vi "Get Functions Path.vi"(8 "error in (no error)":errorcluster) -> (0 "error out":errorcluster, 3 "Function List":path)   [LabVIEW 2016, in "scripts manager.lvclass"]
uses:
  scripts manager.lvclass
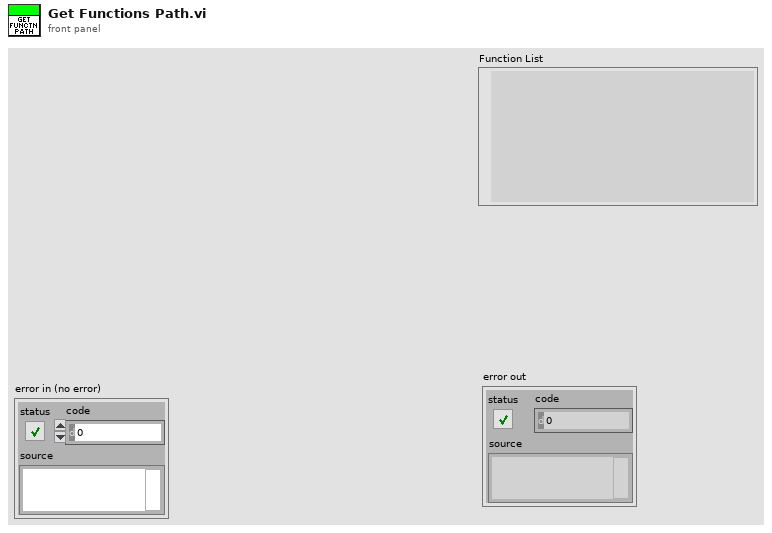
[diagram p1: front panel]
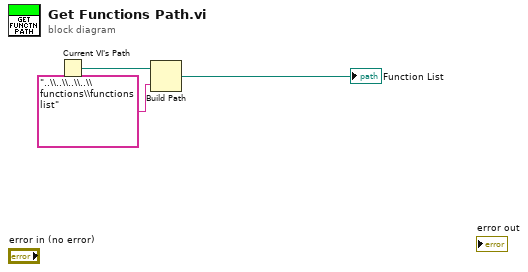
[diagram p0: block diagram]
diagram:
  n1 = Current VI's Path() -> (path=w3:path)
  n2 = Build Path(base path=w3, name or relative path="..\\..\\..\\..\\functions\\functions list") -> (appended path=→"Function List":path)
